vi "StopSecondary.vi"   [LabVIEW 2019]
uses:
  Controls/Ball System Actions.ctl
  Controls/Lift System Actions.ctl
  Controls/Spinner Actions.ctl
types:
  T1 = typedef "Spinner Actions.ctl" = cluster{"Manual Mode ":bool, "Auto rotate n times":bool, "Auto rotate to color\t":bool, "Extend and Retract Arm\t":bool, "Manual Rotation Speed":dbl}
  T2 = typedef "Lift System Actions.ctl" = cluster{"Arm Deploy Piston":bool, "Enable Lift Arm":bool, "Enable Climber":bool, "Climber Velocity":dbl, "Lift Arm Velocity":dbl}
  T3 = typedef "Ball System Actions.ctl" = cluster{"Intake Piston ":bool, "Shoot Ball":bool, "Tube up one Increment\t":bool, "Reverse Ball Intake":bool, "Tube Piston":bool, "Enable Manual Tube":bool, "Tube up four Increments":bool, "Manual Tube Velocity":dbl, "Ball Intake Speed":dbl, "Color Wheel (Shooter)":bool, "Reverse Shooter":bool}
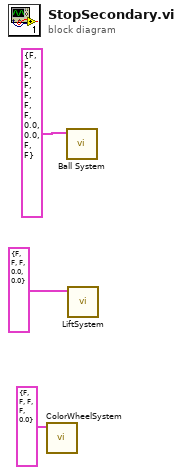
[diagram p0: block diagram]
diagram:
  n1 = call "ColorWheelSystem.vi"("SpinnerActions"=T1 {"Manual Mode "=FALSE, "Auto rotate n times"=FALSE, "Auto rotate to color\t"=FALSE, "Extend and Retract Arm\t"=FALSE, "Manual Rotation Speed"=0.0}) -> ()  [unwired: 11 in]
  n2 = call "Ball System.vi"("Ball System Actions"=T3 {"Intake Piston "=FALSE, "Shoot Ball"=FALSE, "Tube up one Increment\t"=FALSE, "Reverse Ball Intake"=FALSE, "Tube Piston"=FALSE, "Enable Manual Tube"=FALSE, "Tube up four Increments"=FALSE, "Manual Tube Velocity"=0.0, "Ball Intake Speed"=0.0, "Color Wheel (Shooter)"=FALSE, "Reverse Shooter"=FALSE}) -> ()  [unwired: 10 in]
  n3 = call "LiftSystem.vi"("Lift System Actions"=T2 {"Arm Deploy Piston"=FALSE, "Enable Lift Arm"=FALSE, "Enable Climber"=FALSE, "Climber Velocity"=0.0, "Lift Arm Velocity"=0.0}) -> ()  [unwired: 11 in]
